vi "VCS Get All Digital Inputs.vi"(8 "error in (no error)":errorcluster, 11 "axis in":cluster{"keyHandle":u32, "nodeId":u16}={"keyHandle"=0, "nodeId"=1}) -> (0 "error out":errorcluster, 2 "digital inputs":u16(ring)=15 items=["Negative Limit Switch"=0, "Positive Limit Switch"=1, "Home Switch"=2, "Position Marker"=3, "Drive Enable"=4, "Quick Stop"=5, "General Purpose A"=15, "General Purpose B"=14, "General Purpose C"=13, "General Purpose D"=12, "General Purpose E"=11, "General Purpose F"=10, "General Purpose G"=9, "General Purpose H"=8, "Reserved A"=7, "Reserved B"=6], 3 "axis out":cluster{"keyHandle":u32, "nodeId":u16}={"keyHandle"=0, "nodeId"=1})   [LabVIEW 2018]
doc: "<B>VCS Get All Digital Inputs</B> returns state of all digital inputs."
uses:
  Resources/EposCmd.dll
  Resources/EposCmd64.dll
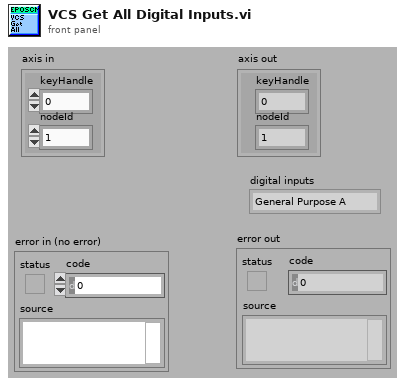
[diagram p1: front panel]
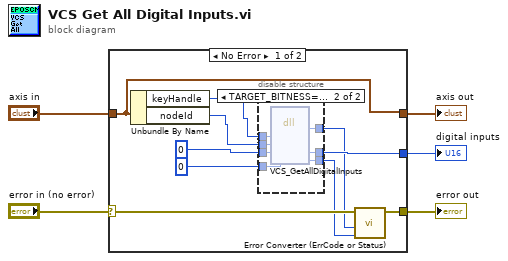
[diagram p0: block diagram]
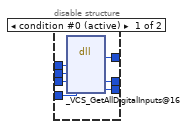
[diagram p2: hidden frame]
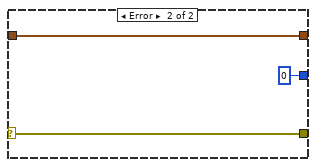
[diagram p3: hidden frame]
diagram:
  n1 = case shown="No Error" "error in (no error)" {
    selector: "error in (no error)" -> [w14 w32]
    tunnel: [w13 w32] -> w4
    tunnel: [w15 u16 0 ("pInputs")] -> w1
    tunnel: "axis in" -> [w7 w31]
    tunnel: [w7 w31] -> w2
    frame No Error {
      n2 = Unbundle By Name(w7) -> ("keyHandle"=w11:u32, "nodeId"=w10:u16)
      n3 = disable-structure shown="TARGET_BITNESS==64" {
        disable-tunnel: [w22 w29] -> w15
        disable-tunnel: [w21 w28] -> w12
        disable-tunnel: w11 -> [w20 w27]
        disable-tunnel: w10 -> [w19 w26]
        disable-tunnel: u16 0 ("pInputs") -> [w18 w25]
        disable-tunnel: u32 0 ("pErrorCode") -> [w17 w24]
        disable-tunnel: [w16 w23] -> w6
        frame condition #0 (active) {
          n4 = dll-call lib="C:/Projeto em LabVIEW/EPOS-LabVIEW-Instrument-Driver-En/LabVIEW/maxon EPOS/Resources/EposCmd.*" fn="_VCS_GetAllDigitalInputs@16"("KeyHandle"=w20, "NodeId"=w19, "pInputs"=w18, "pErrorCode"=w17) -> (w16:i32, "pInputs"=w22:u16, "pErrorCode"=w21:u32)  [unwired: 5 in, 2 out]
        }
        frame condition #1 {
          n5 = dll-call lib="C:/setup/Resources/EposCmd64.*" fn="VCS_GetAllDigitalInputs" ("EposCmd.dll:_VCS_GetAllDigitalInputs@16")("KeyHandle"=w27, "NodeId"=w26, "pInputs"=w25, "pErrorCode"=w24) -> ("Rückgabetyp"=w23:i32, "pInputs"=w29:u16, "pErrorCode"=w28:u32)  [unwired: 5 in, 2 out]
        }
      }
      n6 = call "Error Converter (ErrCode or Status).vi"("error code"=w12, "return type"=w6, "error in (no error)"=w14) -> ("error out"=w13:errorcluster)  [unwired: 7 in]
    }
    frame Error {
    }
  }
  "error out" <- w4
  "axis out" <- w2
  "digital inputs" <- w1
